vi "Apply Settings.vi"(8 "error in (no error)":errorcluster, 10 "User Project":refnum<vi>, 11 "MeasurementMetaData in":refnum<class "MeasurementMetaData.lvclass">) -> (0 "error out":errorcluster, 3 "MeasurementMetaData out":refnum<class "MeasurementMetaData.lvclass">)   [LabVIEW 2016, in "MeasurementMetaData.lvclass"]
uses:
  MeasurementMetaData.lvclass
  C:/Program Files (x86)/National Instruments/LabVIEW 2016/resource/dialog/NewProjectWizard/MetaDataObj/MetaDataObj.lvclass
  MeasurementMetaData.lvclass/MeasurementMetaData.ctl
  <resource>/dialog/NewProjectWizard/MetaDataObj/MetaDataObj.lvclass
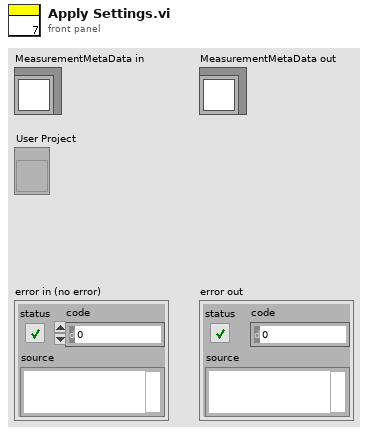
[diagram p1: front panel]
types:
  T1 = typedef "MeasurementMetaData.lvclass/Plugin Settings.ctl" = cluster{"Override Configure Method":bool, "Generate Custom Results Object":bool, "Override Measure Method":bool, "Override Close Method":bool, "Scope?":bool, "DMM?":bool, "FGEN?":bool, "PSU?":bool, "Acquisition Mode":enum16{"Continuous", "Single-Shot"}}
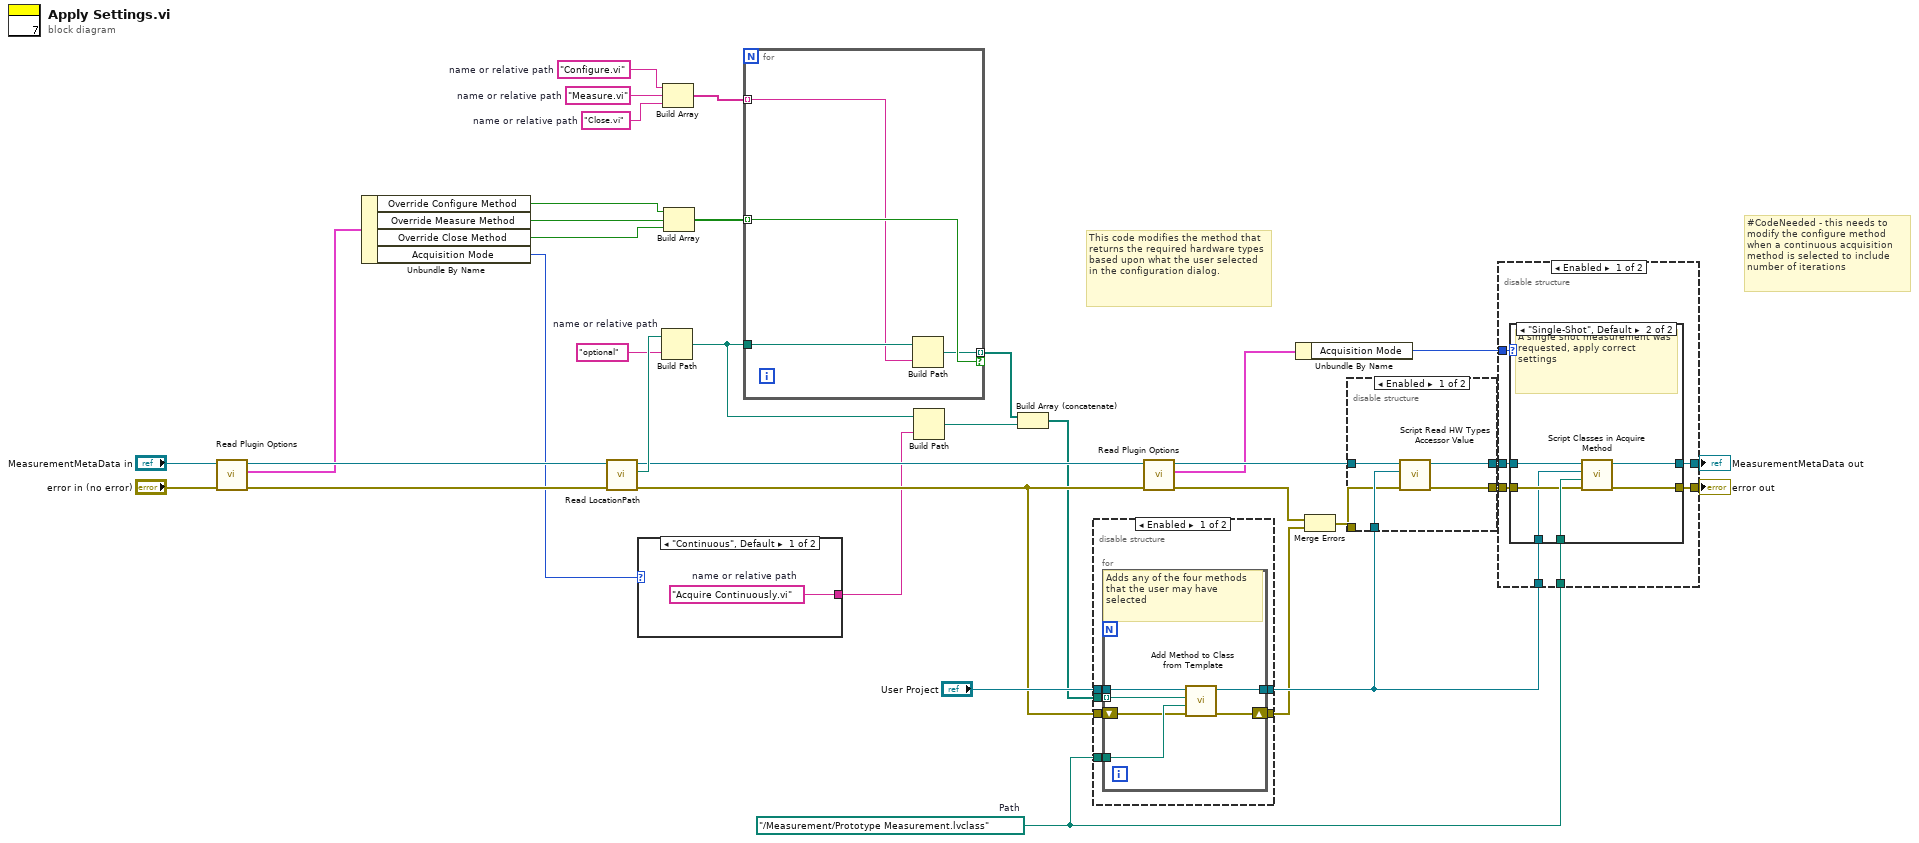
[diagram p0: block diagram]
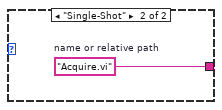
[diagram p6: hidden frame]
diagram:
  w8 = "Close.vi"  # name or relative path
  w31 = "Configure.vi"  # name or relative path
  w9 = "Measure.vi"  # name or relative path
  w26 = "optional"  # name or relative path
  w23 = path "../Measurement/Prototype Measurement.lvclass"  # Path
  # "#CodeNeeded - this needs to \nmodify the configure method\nwhen a continuous acquisition\nmethod is selected to include\nnumber of iterations"
  # "This code modifies the method that returns the required hardware types based upon what the user selected in the configuration dialog."
  n1 = call "Read Plugin Options.vi"("error in (no error)"="error in (no error)", "MeasurementMetaData in"="MeasurementMetaData in") -> ("error out"=w34:errorcluster, "Plugin Options"=w5:T1, "MeasurementMetaData out"=w33:refnum<class "MeasurementMetaData.lvclass">)  [unwired: 7 in]
  n2 = Unbundle By Name "Unbundle By Name"(w5) -> ("Override Configure Method"=w29:bool, "Override Measure Method"=w28:bool, "Override Close Method"=w27:bool, "Acquisition Mode"=w1:enum16{"Continuous", "Single-Shot"})
  n3 = call <resource>:"Read LocationPath.vi"("error in (no error)"=w34, "MetaDataObj in"=w33) -> ("error out"=w13:errorcluster, "LocationPath"=w35:path, "MetaDataObj out"=w17:refnum<class "MeasurementMetaData.lvclass">)  [unwired: 7 in]
  n4 = case shown="\"Continuous\", Default" w1 {
    tunnel: [w37 w38] -> w3
    frame "Continuous", Default {
      w37 = "Acquire Continuously.vi"  # name or relative path
    }
    frame "Single-Shot" {
      w38 = "Acquire.vi"  # name or relative path
    }
  }
  n5 = Build Path(base path=w35, name or relative path=w26) -> (appended path=w4:path)
  n6 = Build Array "Build Array"(w31, w9, w8) -> (w32:string[])
  n7 = Build Array "Build Array"(w29, w28, w27) -> (w30:bool[])
  n8 = for {
    tunnel: w30 -> [w42] mode=indexing
    tunnel: w32 -> [w39] mode=indexing
    tunnel: [w40] -> w7 mode=indexing if=w42
    tunnel: w4 -> [w41]
    n9 = Build Path(base path=w41, name or relative path=w39) -> (appended path=w40:path)
  }
  n10 = Build Path(base path=w4, name or relative path=w3) -> (appended path=w2:path)
  n11 = Build Array (concatenate)(w7, w2) -> (w6:path[])
  n12 = disable-structure shown="Enabled" {
    disable-tunnel: "User Project" -> [w48 w55]
    disable-tunnel: w23 -> [w47 _]
    disable-tunnel: [w46 w55] -> w18
    disable-tunnel: w13 -> [w45 _]
    disable-tunnel: [w44 _] -> w10
    disable-tunnel: w6 -> [w43 _]
    frame Enabled {
      n13 = for {
        tunnel: w47 -> [w54]
        tunnel: w48 -> [w53]
        tunnel: [w52] -> w46
        tunnel: w43 -> [w51] mode=indexing
        shift-right: [w50] -> w44
        shift-left: w45 -> [w49]
        # "Adds any of the four methods that the user may have selected"
        n14 = call "Add Method to Class from Template.vi"("error in (no error)"=w49, "Path to Class"=w54, "Location of Template"=w51, "Project in"=w53) -> ("error out"=w50:errorcluster, "Project out"=w52:refnum<vi>)  [unwired: 6 in]
      }
    }
    frame Disabled {
    }
  }
  n15 = call "Read Plugin Options.vi"("error in (no error)"=w13, "MeasurementMetaData in"=w17) -> ("error out"=w12:errorcluster, "Plugin Options"=w14:T1, "MeasurementMetaData out"=w16:refnum<class "MeasurementMetaData.lvclass">)  [unwired: 7 in]
  n16 = Unbundle By Name "Unbundle By Name"(w14) -> ("Acquisition Mode"=w15:enum16{"Continuous", "Single-Shot"})
  n17 = Merge Errors(w12, w10) -> (w11:errorcluster)
  n18 = disable-structure shown="Enabled" {
    disable-tunnel: [w60 w61] -> w22
    disable-tunnel: [w59 _] -> w21
    disable-tunnel: w18 -> [w58 _]
    disable-tunnel: w16 -> [w57 w61]
    disable-tunnel: w11 -> [w56 _]
    frame Enabled {
      n19 = call "Script Read HW Types Accessor Value.vi"("error in (no error)"=w56, "Project in"=w58, "MeasurementMetaData in"=w57) -> ("error out"=w59:errorcluster, "MeasurementMetaData out"=w60:refnum<class "MeasurementMetaData.lvclass">)  [unwired: 7 in]
    }
    frame Disabled {
    }
  }
  n20 = disable-structure shown="Enabled" {
    disable-tunnel: w23 -> [w68 _]
    disable-tunnel: w22 -> [w67 w78]
    disable-tunnel: w21 -> [w66 w77]
    disable-tunnel: [w65 w78] -> w20
    disable-tunnel: [w64 w77] -> w19
    disable-tunnel: w18 -> [w63 _]
    disable-tunnel: w15 -> [w62 _]
    frame Enabled {
      n21 = case shown="\"Single-Shot\", Default" w62 {
        tunnel: w68 -> [_ w76]
        tunnel: w67 -> [w69 w75]
        tunnel: w66 -> [w70 w74]
        tunnel: [w69 w73] -> w65
        tunnel: [w70 w72] -> w64
        tunnel: w63 -> [_ w71]
        frame "Continuous" {
          # "A continously running measurement was requested, apply correct settings"
        }
        frame "Single-Shot", Default {
          # "A single shot measurement was requested, apply correct settings"
          n22 = call "Script Classes in Acquire Method.vi"("error in (no error)"=w74, "Path"=w76, "Project in"=w71, "MeasurementMetaData in"=w75) -> ("error out"=w72:errorcluster, "MeasurementMetaData out"=w73:refnum<class "MeasurementMetaData.lvclass">)  [unwired: 6 in]
        }
      }
    }
    frame Disabled {
    }
  }
  "error out" <- w19
  "MeasurementMetaData out" <- w20
